vi "LoadModel.vi"(8 "error in (no error)":errorcluster, 10 "Actor In":refnum<class "Actor.lvclass">, 11 "GRMActor in":refnum<class "CameraController.lvclass">) -> (0 "error out":errorcluster, 3 "GRMActor out":refnum<class "CameraController.lvclass">)   [LabVIEW 2020, in "CameraController.lvlib" / "CameraController.lvclass"]
uses:
  CameraController.lvclass
  <vilib>/ActorFramework/Actor/Actor.lvclass
  Model/Hardware Layer/Simulation Hardware/DemoCamera/DemoCamera/DemoCamera.lvclass
  D:/Daguan/Development/MMicroscopyFramework/Model/Hardware Abstraction Layer/Component/Camera/Camera/Camera.lvclass
  Model/Hardware Layer/Real Hardware/Camera_Prime95B/Camera_Prime95B/Camera_Prime95B.lvclass
  CameraController.lvclass/CameraController.ctl
  Model/Hardware Abstraction Layer/Component/Camera/Camera/Camera.lvclass
  C:/Program Files/National Instruments/LabVIEW 2020/vi.lib/ActorFramework/Actor/Actor.lvclass
  Model/Hardware Abstraction Layer/Component/GenericActor/GenericActor/GenericController.lvclass
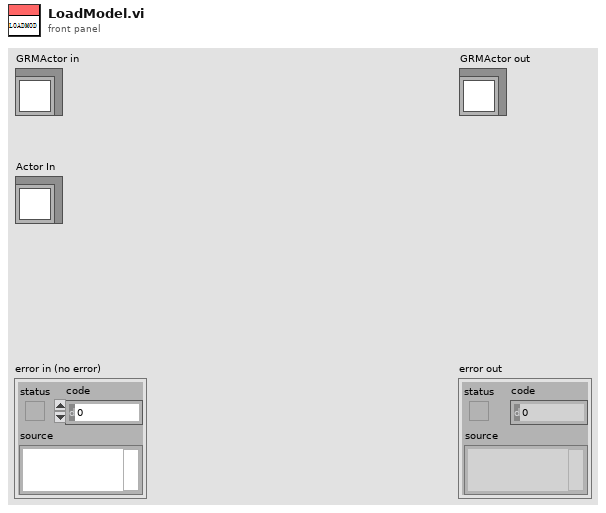
[diagram p1: front panel]
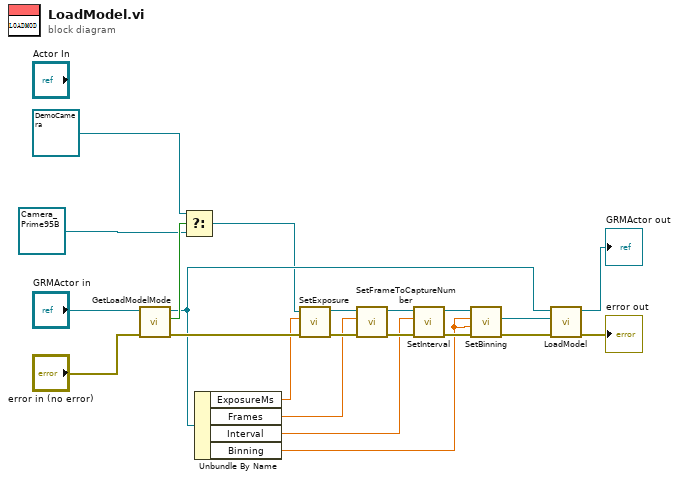
[diagram p0: block diagram]
diagram:
  n1 = call-dynamic "GetLoadModelMode.vi"("error in (no error)"="error in (no error)", "GenericController in"="GRMActor in") -> ("error out"=w19:errorcluster, "LoadDemoModel"=w17:bool, "GenericController out"=w12:refnum<class "CameraController.lvclass">)  [unwired: 7 in]
  n2 = Select(t=refnum<class "DemoCamera.lvclass"> refnum ("DemoCamera.lvlib:DemoCamera.lvclass"), s=w17, f=refnum<class "Camera_Prime95B.lvclass"> refnum ("Camera_Prime95B.lvlib:Camera_Prime95B.lvclass")) -> (s? t:f=w10:refnum<class "Camera.lvclass">)
  n3 = Unbundle By Name(w12) -> ("ExposureMs"=w9:dbl, "Frames"=w6:dbl, "Interval"=w2:dbl, "Binning"=w1:dbl)
  n4 = call-dynamic "SetExposure.vi"("error in (no error)"=w19, "Setting.Exposure"=w9, "Camera in"=w10) -> ("error out"=w11:errorcluster, "Camera out"=w7:refnum<class "Camera.lvclass">)  [unwired: 7 in]
  n5 = call-dynamic "SetFrameToCaptureNumber.vi"("error in (no error)"=w11, "Setting.FramesToCapture"=w6, "Camera in"=w7) -> ("error out"=w8:errorcluster, "Camera out"=w4:refnum<class "Camera.lvclass">)  [unwired: 7 in]
  n6 = call-dynamic "SetInterval.vi"("error in (no error)"=w8, "Setting.Interval"=w2, "Camera in"=w4) -> ("error out"=w5:errorcluster, "Camera out"=w3:refnum<class "Camera.lvclass">)  [unwired: 7 in]
  n7 = call-dynamic "SetBinning.vi"("error in (no error)"=w5, "Setting.Binning.BinY"=w1, "Setting.Binning.BinX"=w1, "Camera in"=w3) -> ("error out"=w14:errorcluster, "Camera out"=w13:refnum<class "Camera.lvclass">)  [unwired: 6 in]
  n8 = call-parent "LoadModel.vi"("error in (no error)"=w14, "Actor In"=w13, "GRMActor in"=w12) -> ("error out"=→"error out":errorcluster, "GRMActor out"=→"GRMActor out":refnum<class "CameraController.lvclass">)  [unwired: 7 in]
